vi "Static Read.vi"(8 "error in (no error)":errorcluster, 11 "Abs_Complex Extended Float in":refnum<class "Abs_Complex Extended Float.lvclass">) -> (0 "error out":errorcluster, 2 "Value":cxt, 3 "Abs_Complex Extended Float out":refnum<class "Abs_Complex Extended Float.lvclass">)   [LabVIEW 2021, in "Abs_Complex Extended Float.lvclass"]
uses:
  Abs_Complex Extended Float.lvclass
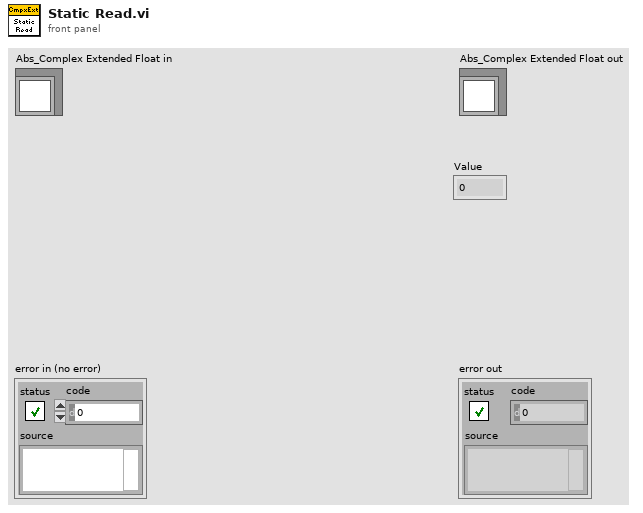
[diagram p1: front panel]
types:
  T1 = typedef "Abs_Complex Extended Float.lvclass/Type.ctl" = cxt
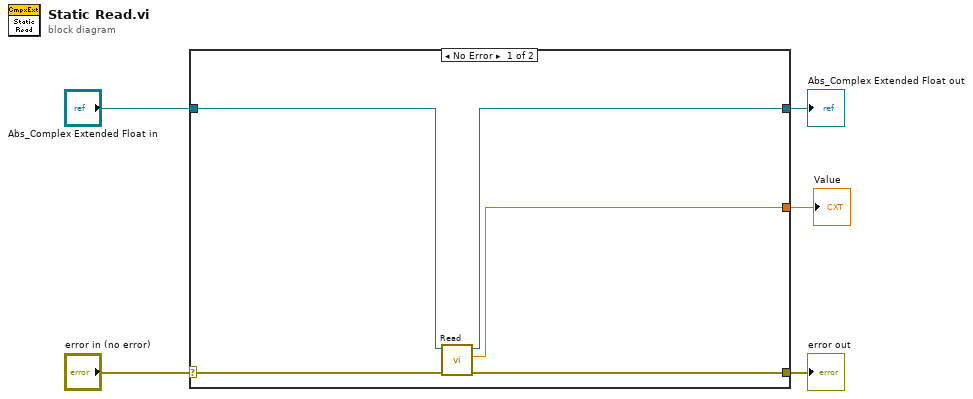
[diagram p0: block diagram]
diagram:
  n1 = case shown="No Error" "error in (no error)" {
    selector: "error in (no error)" -> [w10 w12]
    tunnel: [w9 w12] -> w4
    tunnel: [w7 w11] -> w2
    tunnel: "Abs_Complex Extended Float in" -> [w8 w11]
    tunnel: [w6 _] -> w1
    frame No Error {
      n2 = call-dynamic "Read.vi"("error in (no error)"=w10, "Double Float.lvclass_340760 in"=w8) -> ("error out"=w9:errorcluster, "Value"=w6:T1, "Double Float.lvclass_340760 out"=w7:refnum<class "Abs_Complex Extended Float.lvclass">)  [unwired: 7 in]
    }
    frame Error {
    }
  }
  "error out" <- w4
  "Abs_Complex Extended Float out" <- w2
  "Value" <- w1
